vi "celsius_to_fahrenheit.vi"(1 "Celcius":sgl format="%#.1f") -> (0 "Fahrenheit":sgl format="%#.1f")   [LabVIEW 2012]
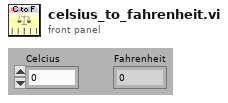
[diagram p1: front panel]
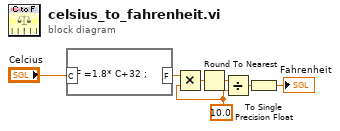
[diagram p0: block diagram]
diagram:
  w4 = 10.0 ("y")
  n1 = formula code="F =1.8* C+32 ;"("C"="Celcius") -> ("F"=w2:dbl)
  n2 = Multiply(x=w2, y=w4) -> (x*y=w6:dbl)
  n3 = Round To Nearest(number=w6) -> (nearest integer value=w5:dbl)
  n4 = Divide(x=w5, y=w4) -> (x/y=w3:dbl)
  n5 = To Single Precision Float(number=w3) -> (single precision float=→"Fahrenheit":sgl)
